vi "is_sweep_done.vi"(8 "error in (no error)":errorcluster, 11 "ExperimentControllerDL090130Interval in":refnum<class "ExperimentControllerDL090130Interval.lvclass">) -> (0 "error out":errorcluster, 2 "sweep done?":bool, 3 "ExperimentControllerDL090130Interval out":refnum<class "ExperimentControllerDL090130Interval.lvclass">)   [LabVIEW 2010, in "ExperimentControllerDL090130Interval.lvclass"]
uses:
  ExperimentControllerDL090130Interval.lvclass
  ExperimentControllerDL090130Interval.lvclass/ExperimentControllerDL090130Interval.ctl
  Sweep/GenericSweep/GenericSweep/GenericSweep.lvclass
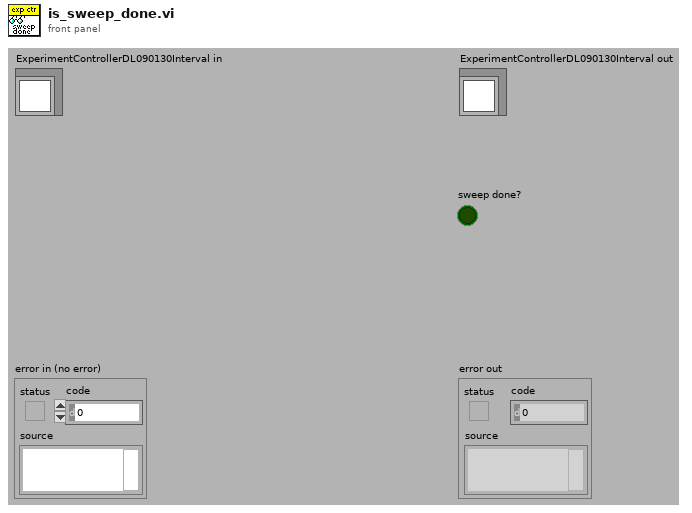
[diagram p1: front panel]
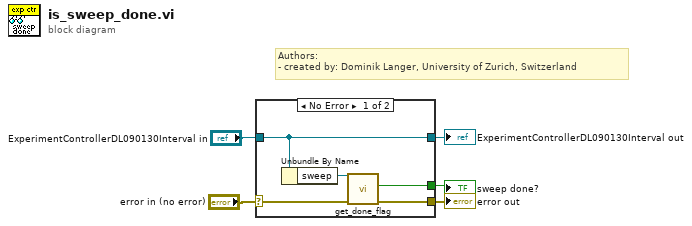
[diagram p0: block diagram]
diagram:
  # "Authors: \n- created by: Dominik Langer, University of Zurich, Switzerland"
  n1 = case shown="No Error" "error in (no error)" {
    selector: "error in (no error)" -> [w9 w12]
    tunnel: [w8 w12] -> w4
    tunnel: [w10 w11] -> w2
    tunnel: "ExperimentControllerDL090130Interval in" -> [w10 w11]
    tunnel: [w6 _] -> w1
    frame No Error {
      n2 = Unbundle By Name(w10) -> ("sweep"=w7:refnum<class "GenericSweep.lvclass">)
      n3 = call-dynamic "get_done_flag.vi"("error in (no error)"=w9, "GenericSweep in"=w7) -> ("error out"=w8:errorcluster, "sweep done?"=w6:bool)  [unwired: 7 in, 1 out]
    }
    frame Error {
    }
  }
  "error out" <- w4
  "ExperimentControllerDL090130Interval out" <- w2
  "sweep done?" <- w1
